vi "Signal Generator.vi"() -> ()   [LabVIEW 2016]
doc: "I. Description:\nThis example demonstrates how to continuously output a waveform using an internal sample clock. The automatic regeneration of data has been disabled, so new data has to be provided throughout the duration of the continuous Analog Output operation. This allows the generation of any arbitrary frequency as this VI computes new data for each iteration of the loop, maintaining phase continuity of the signal. The regeneration of data has also been adjusted so that the newest data is output as quickly as possible; thus reducing the lag between the changing of the data and the output of that data.\n\nII. Instructions for Running:\n1. Select the Physical Channel to correspond to where your signal is output on the DAQ device.\n2. Enter the Minimum and Maximum Voltage range.\n3. Specify the desired Sample Clock Rate of the output Waveform. Higher sample clock rates will produce a smoother waveform.\n4. Manually specify the Analog Output buffer size, in number of samples. A larger buffer would help non-regenerative operations avoid errors due to occasional high CPU load. \nNote: \nThe Analog Output buffer has to be at least as big as the amount of data being written to the board per iteration. The recommended buffer size would be at least twice the amount of data being written to the board per iteration.\n5. Enter the Waveform Information. See the documentation of the Basic Function Generator SubVI for information on each parameter.\n\nIII. Block Diagram Steps:\n1. Create an Analog Output Voltage channel.\n2. Configure the task to prohibit the automatic regeneration of data.\n2a. Set the transfer condition to Less than Full. Allows for more rapid updates of Output Buffer.\n3. Call the DAQmx (Sample Clock) VI to set the sample clock rate. Additionally, set the sample mode to Continuous.\n4. Read the actual sample clock rate (eventually coerced depending on the hardware used). \n5. Compute the desired waveform, using the buffer size and the actual update rate. This VI keeps track of the phase of the waveform to ensure that the generated signal is continuous.\n6. Write the waveform to the output buffer. \n7a. Call the Start VI. This is only needed when the loop is executed for the first time.\n7b. Do nothing.\n8. Loop continuously until user presses the Stop button. Every iteration computes and writes a new waveform to the buffer.\n9. Call the Clear Task VI to clear the Task.\n10. Use the popup dialog box to display an error or warning if any.\n\nIV. I/O Connections Overview:\nMake sure your signal output terminal matches the Physical Channel I/O Control. For further connection information, refer to your hardware reference manual."
uses:
  <vilib>/Utility/error.llb/DialogType.ctl
  <vilib>/DAQmx/write.llb/DAQmx Write.vi
  <vilib>/DAQmx/create/channels.llb/DAQmx Create Virtual Channel.vi
  <vilib>/DAQmx/configure/timing.llb/DAQmx Timing.vi
  <vilib>/DAQmx/miscellaneous.llb/DAQmx Fill In Error Info.vi
  <vilib>/measure/NI_MABase.lvlib
  <resource>/objmgr/daqmx.rc
panel:
  in  "Offset":dbl=0.1 format="%0.2p"
  in  "Size (Samples)":u32=1000000
  out "Actual Sample Clock Rate":dbl=20000.0 format="%.2f"
  in  "Sample Clock Rate":dbl=100000.0 format="%0.2f"
  in  "Waveform Type":T1(ring)
  in  "Frequency":dbl=1.0 min=0.0 max=100.0 step=1.0 format="%.2f"
  in  "Amplitude":dbl=0.1 format="%0.2p"
  out "Waveform Graph":waveform(dbl)(graph)={"t0"=timestamp(12.75 s since 1904-01-01), "dt"=5e-05, "Y"=[]} caption="Output Waveform"
  in  "Physical Channels":tag="DAQ/ao0"
  in  "Minimum Value":dbl=-1.0 min=-5.0 max=0.0 step=0.001 format="%0.2f"
  in  "Maximum Value":dbl=1.0 min=0.0 max=5.0 step=0.001 format="%0.2f"
  in  "stop":bool
  # "Channel Parameters"
  # "Timing Parameters"
  # "Buffer Parameters"
  # "Waveform Information"
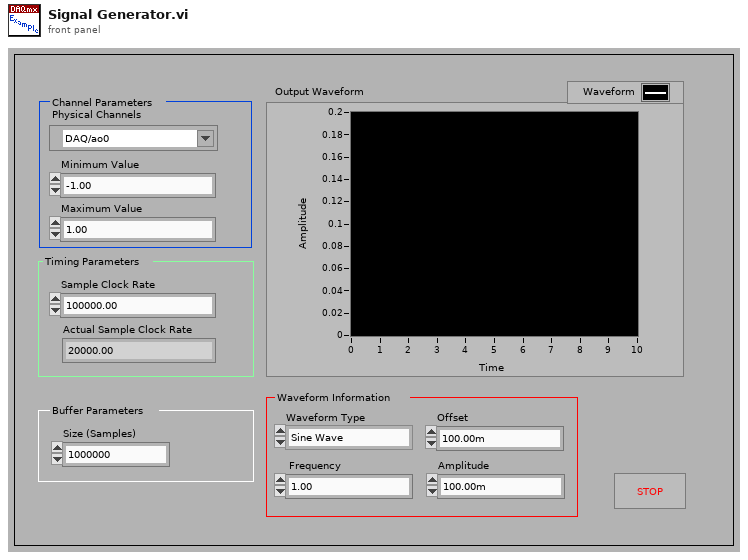
[diagram p1: front panel]
types:
  T1 = enum16{"Sine Wave", "Triangle Wave", "Square Wave", "Sawtooth Wave"}
  T2 = typedef "DialogType.ctl" = u16
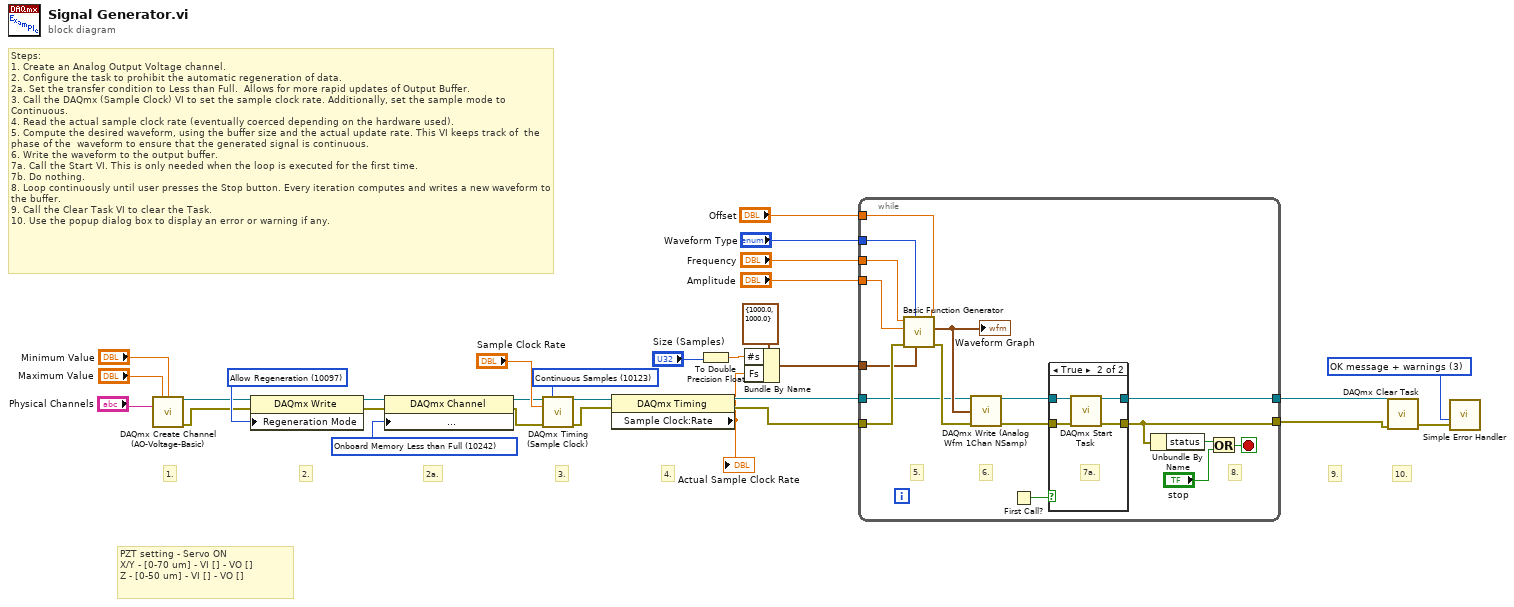
[diagram p0: block diagram]
diagram:
  w7 = 10242 items=["Onboard Memory Empty"=10235, "Onboard Memory Half Full or Less"=10239, "Onboard Memory Less than Full"=10242] ("AO.DataXferReqCond")
  w17 = 10097 items=["Allow Regeneration"=10097, "Do Not Allow Regeneration"=10158] ("RegenMode")
  w25 = T2 3 items=["no dialog", "OK message", "continue or stop message", "OK message + warnings", "continue/stop + warnings"] ("type of dialog (OK msg:1)")
  w29 = 10123 items=["Finite Samples"=10178, "Continuous Samples"=10123] ("sample mode")
  # "PZT setting - Servo ON\nX/Y - [0-70 um] - VI [] - VO [] \nZ - [0-50 um] - VI [] - VO []"
  # "2a."
  # "4."
  # "3."
  # "Steps:\n1. Create an Analog Output Voltage channel.\n2. Configure the task to prohibit the automatic regeneration of data.\n2a. Set the transfer condition to Less than Full.  Allows for more rapid updates of Output Buffer. \n3. Call the DAQmx (Sample Clock) VI to set the sample clock rate. Additionally, set the sample mode to Continuous.\n4. Read the actual sample clock rate (eventually coerced depending on the hardware used).\n5. Compute the desired waveform, using the buffer size and the actual update rate. This VI keeps track of  the phase of the  waveform to ensure that the generated signal is continuous.\n6. Write the waveform to the output buffer. \n7a. Call the Start VI. This is only needed when the loop is executed for the first time.\n7b. Do nothing.\n8. Loop continuously until user presses the Stop button. Every iteration computes and writes a new waveform to the buffer.\n9. Call the Clear Task VI to clear the Task.\n10. Use the popup dialog box to display an error or warning if any."
  # "10."
  # "9."
  # "2."
  # "1."
  n1 = call-poly <vilib>:"DAQmx Create Channel (AO-Voltage-Basic).vi"("maximum value"="Maximum Value", "minimum value"="Minimum Value", "physical channels"="Physical Channels") -> ("task out"=w16:refnum<k21>, "error out"=w15:errorcluster)  [unwired: 11 in]
  n2 = property class="DAQmx Write"(reference=w16, error in=w15, "Regeneration Mode"=w17) -> (reference out=w11:refnum<k21>, error out=w8:errorcluster)
  n3 = property class="DAQmx Channel"(reference=w11, error in=w8, "Analog Output:General Properties:Advanced:Data Transfer and Memory:Data Transfer Request Condition"=w7) -> (reference out=w10:refnum<k21>, error out=w9:errorcluster)
  n4 = call-poly <vilib>:"DAQmx Timing (Sample Clock).vi"("task/channels in"=w10, "sample mode"=w29, "rate"="Sample Clock Rate", "error in"=w9) -> ("task out"=w22:refnum<k21>, "error out"=w21:errorcluster)  [unwired: 10 in]
  n5 = property class="DAQmx Timing"(reference=w22, error in=w21) -> (reference out=w5:refnum<k21>, error out=w4:errorcluster, "Sample Clock:Rate"=w2:dbl)
  "Actual Sample Clock Rate" <- w2
  n6 = To Double Precision Float(number="Size (Samples)") -> (double precision float=w12:dbl)
  n7 = Bundle By Name(cluster=cluster{"Fs":dbl, "#s":dbl} {"Fs"=1000.0, "#s"=1000.0} ("sampling info"), "#s"=w12, "Fs"=w2) -> (w6:cluster{"Fs":dbl, "#s":dbl})
  n8 = while {
    tunnel: w5 -> [w37]
    tunnel: [w33] -> w24
    tunnel: w4 -> [w44]
    tunnel: [w34] -> w3
    tunnel: "Waveform Type" -> [w42]
    tunnel: "Frequency" -> [w41]
    tunnel: "Amplitude" -> [w40]
    tunnel: w6 -> [w39]
    tunnel: "Offset" -> [w31]
    stop <- w47 stop-if-true
    # "8."
    # "6."
    # "5."
    n9 = call <vilib>:"Basic Function Generator.vi"("offset"=w31, "sampling info"=w39, "signal type"=w42, "error in (no error)"=w44, "amplitude"=w40, "frequency"=w41) -> ("error out"=w43:errorcluster, "signal out"=w38:waveform(dbl))  [unwired: 3 in, 1 out]
    "Waveform Graph" <- w38
    n10 = call-poly <vilib>:"DAQmx Write (Analog Wfm 1Chan NSamp).vi"("task/channels in"=w37, "data"=w38, "error in"=w43) -> ("task out"=w36:refnum<k21>, "error out"=w35:errorcluster)  [unwired: 10 in, 1 out]
    n11 = First Call?() -> (First Call?: T/F=w32:bool)
    n12 = case shown="True" w32 {
      tunnel: w36 -> [w49 w53]
      tunnel: w35 -> [w48 w52]
      tunnel: [w48 w51] -> w34
      tunnel: [w49 w50] -> w33
      frame False {
        # "7b."
      }
      frame True {
        # "7a."
        n13 = call <vilib>:"DAQmx Start Task.vi"("task/channels in"=w53, "error in"=w52) -> ("task out"=w50:refnum<k21>, "error out"=w51:errorcluster)  [unwired: 12 in]
      }
    }
    n14 = Unbundle By Name(w34) -> ("status"=w46:bool)
    n15 = Or(x=w46, y="stop") -> (x .or. y?=w47:bool)
  }
  n16 = call <vilib>:"DAQmx Clear Task.vi"("task in"=w24, "error in"=w3) -> ("error out"=w30:errorcluster)  [unwired: 13 in]
  n17 = call <vilib>:"Simple Error Handler.vi"("type of dialog (OK msg:1)"=w25, "error in (no error)"=w30) -> ()  [unwired: 3 in, 5 out]
